vi "Write discovers channels dynamically.vi"(8 "error in":errorcluster, 10 "discovers channels dynamically":bool, 11 "DecideProjectFeatures in":refnum<class "TagBusConfigurablePluginDecideFeatures.lvclass">) -> (0 "error out":errorcluster, 3 "DecideProjectFeatures out":refnum<class "TagBusConfigurablePluginDecideFeatures.lvclass">)   [LabVIEW 2013, in "TagBusConfigurablePluginDecideFeatures.lvclass"]
uses:
  TagBusConfigurablePluginDecideFeatures.lvclass
  TagBusConfigurablePluginDecideFeatures.lvclass/TagBusConfigurablePluginDecideFeatures.ctl
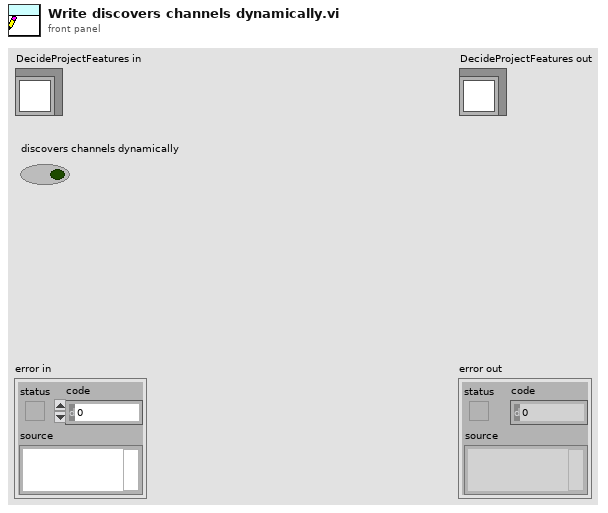
[diagram p1: front panel]
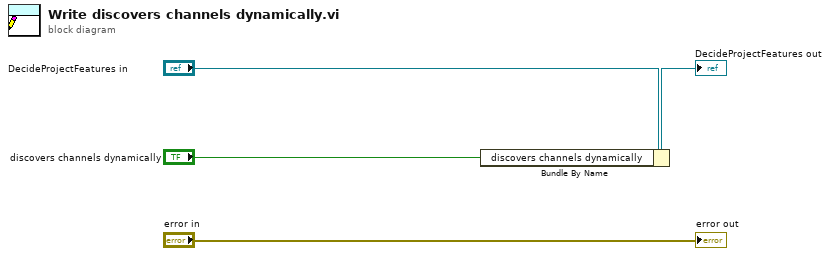
[diagram p0: block diagram]
diagram:
  n1 = Bundle By Name(cluster="DecideProjectFeatures in", "discovers channels dynamically"="discovers channels dynamically") -> (→"DecideProjectFeatures out":refnum<class "TagBusConfigurablePluginDecideFeatures.lvclass">)
  "error out" <- "error in"
